vi "Read Base name.vi"(8 "error in (no error)":errorcluster, 11 "Check Size Message in":refnum<class "Manage File Request.lvclass">) -> (0 "error out":errorcluster, 2 "Base name":string, 3 "Check Size Message out":refnum<class "Manage File Request.lvclass">)   [LabVIEW 2020, in "AIM ARINC 664 Engine.lvlib" / "Implementation.lvlib" / "Frame Logging.lvlib" / "Manage File Request.lvclass"]
uses:
  Manage File Request.lvclass
  Manage File Request.lvclass/Manage File Request.ctl
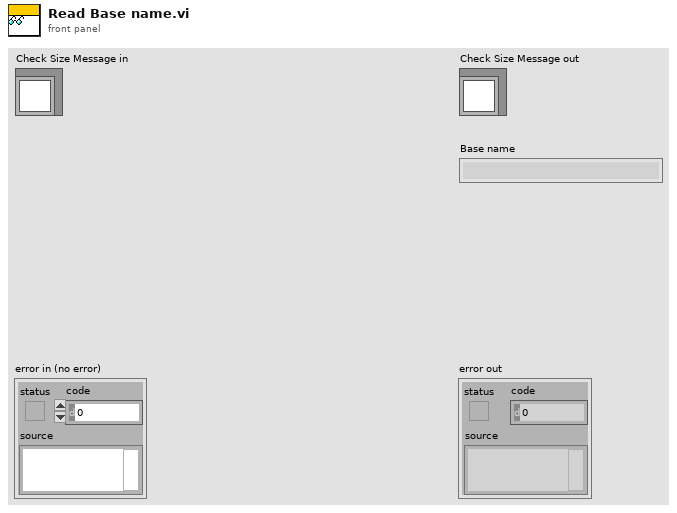
[diagram p1: front panel]
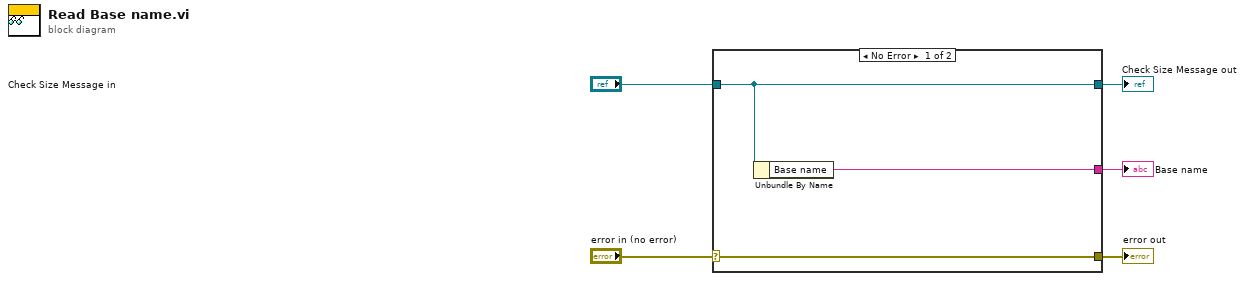
[diagram p0: block diagram]
diagram:
  n1 = case shown="No Error" "error in (no error)" {
    selector: "error in (no error)" -> [w8 w9]
    tunnel: [w8 w9] -> w4
    tunnel: [w7 w10] -> w2
    tunnel: "Check Size Message in" -> [w7 w10]
    tunnel: [w6 _] -> w1
    frame No Error {
      n2 = Unbundle By Name(w7) -> ("Base name"=w6:string)
    }
    frame Error {
    }
  }
  "error out" <- w4
  "Check Size Message out" <- w2
  "Base name" <- w1
